vi "set_DSC_p.vi"(0 "MoAgSy_Host":refnum<class "MoAgSy_Host.lvclass">, 2 "DSC":T1, 5 "error in (no error)":errorcluster) -> (14 "dup MoAgSy_Host":refnum<class "MoAgSy_Host.lvclass">, 19 "error out":errorcluster)   [LabVIEW 2009, in "MoAgSy.lvlib" / "MoAgSy_Host.lvclass"]
doc: "<B>protected</B> VI sets DSC settings of mobile agent base class.\nIs called by public set DSC VI once in the init process of an host vi.\n\nF.Berck@gsi.de\nGSI Darmstadt 2009"
uses:
  MoAgSy_Host.lvclass
  HGF_BaseClasses/HGF_Event/HGF_Event.lvclass
  HGF_BaseClasses/HGF_TriggeredEvent/HGF_TriggeredEvent.lvclass
  HGF_BaseClasses/HGF_Reference/HGF_Reference.lvclass
  MoAgSy_Host.lvclass/MoAgSy_Host.ctl
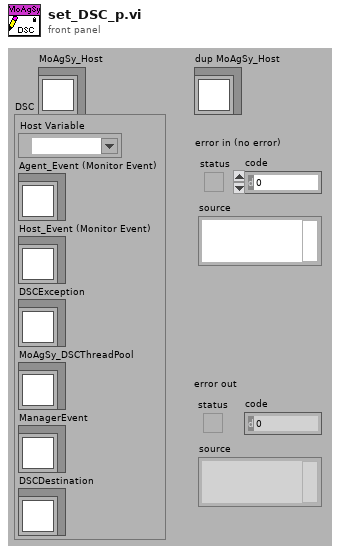
[diagram p1: front panel]
types:
  T1 = cluster{"Host Variable":refnum<k21>, "Agent_Event (Monitor Event)":refnum<class "HGF_Event.lvclass">, "Host_Event (Monitor Event)":refnum<class "HGF_Event.lvclass">, "DSCException":refnum<class "HGF_TriggeredEvent.lvclass">, "MoAgSy_DSCThreadPool":refnum<class "HGF_Reference.lvclass">, "ManagerEvent":refnum<class "HGF_Event.lvclass">, "DSCDestination":refnum<class "HGF_TriggeredEvent.lvclass">}
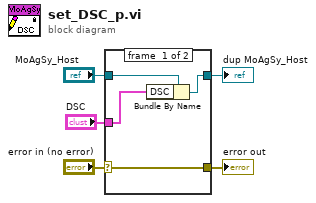
[diagram p0: block diagram]
diagram:
  n1 = case shown="No Error" "error in (no error)" {
    selector: "error in (no error)" -> [w9 w11]
    tunnel: [w9 w11] -> w4
    tunnel: [w7 w10] -> w2
    tunnel: "MoAgSy_Host" -> [w8 w10]
    tunnel: "DSC" -> [w6 _]
    frame #0 {
      n2 = Bundle By Name(cluster=w8, "DSC"=w6) -> (w7:refnum<class "MoAgSy_Host.lvclass">)
    }
    frame #1 {
    }
  }
  "error out" <- w4
  "dup MoAgSy_Host" <- w2
